vi "Create Sprite Points.vi"(4 "Scale":cluster{"X":sgl, "Y":sgl, "Z":sgl}, 5 "Sprite Type":T1=enum."Empty Square", 6 "Vertex Array":cluster{"X":sgl, "Y":sgl, "Z":sgl}[](array[cluster]), 7 "Point Size":sgl, 8 "error in (no error)":errorcluster, 9 "Index Array":i32[](array[numeric]), 10 "Color Array":cluster{"R":sgl, "G":sgl, "B":sgl, "A":sgl}[](array[cluster]), 11 "Dot Object In":refnum<vi>) -> (0 "error out":errorcluster, 3 "Dot Object Out":refnum<vi>)   [LabVIEW 2020, in "3D Plot.lvclass"]
uses:
  3D Plot.lvclass
  Sprite Type.ctl
  LV3DPointTypeDef.ctl
  NI_3D Picture Control.lvlib
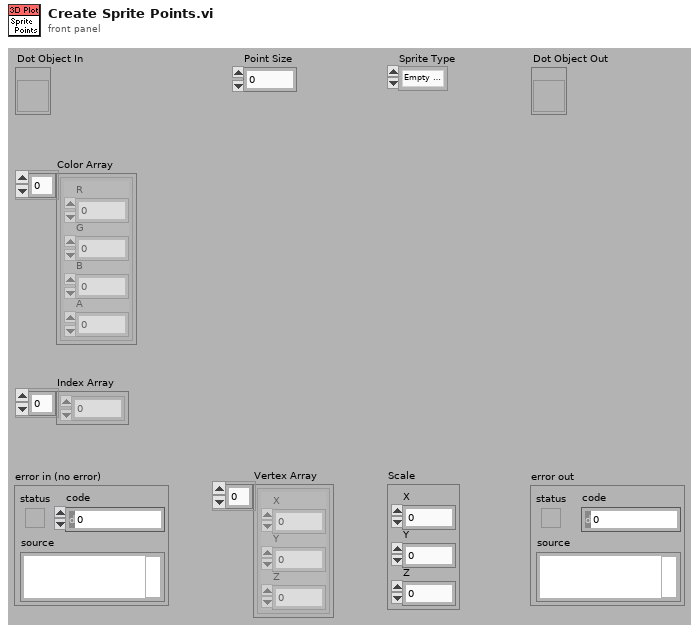
[diagram p1: front panel]
types:
  T1 = typedef "3D Plot.lvclass/Sprite Type.ctl" = enum16{"None", "Empty Square", "Solid Square", "Empty Diamond", "Solid Diamond", "Empty Circle", "Solid Circle", "Asterisk", "Bold X", "Wireframe Sphere", "Solid Sphere", "Wireframe Cube", "Solid Cube"}
  T2 = typedef "LV3DPointTypeDef.ctl" = cluster{"X":sgl, "Y":sgl, "Z":sgl}
  T3 = enum16{"Inherit Value", "Points", "Wireframe", "Polygons"}
  T4 = enum16{"Overall", "Per Primitive", "Per Vertex", "Binding Off"}
  T5 = enum16{"Points", "Lines", "Line Strip", "Line Loop", "Triangles", "Triangle Strip", "Triangle Fan", "Quads", "Quad Strip", "Polygon"}
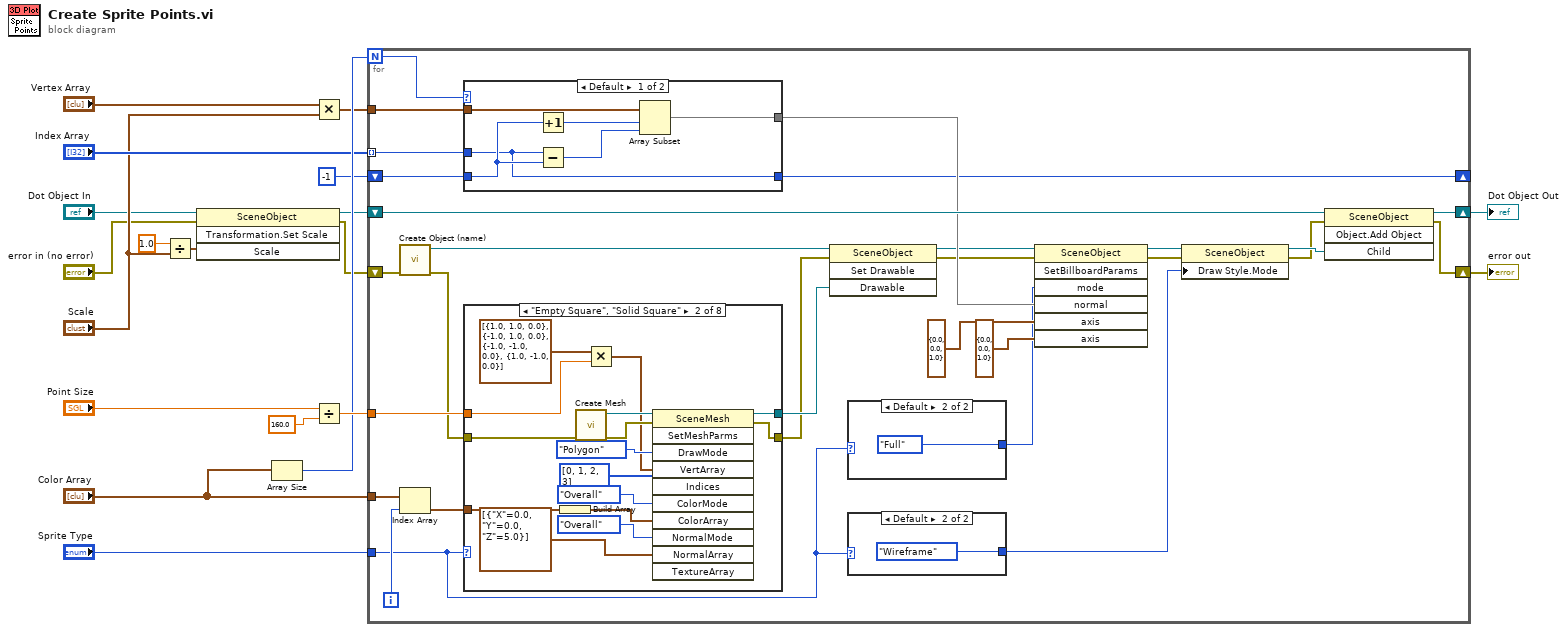
[diagram p0: block diagram]
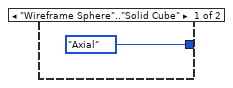
[diagram p2: hidden frame]
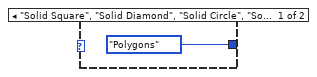
[diagram p4: hidden frame]
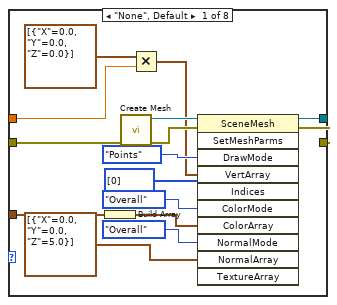
[diagram p5: hidden frame]
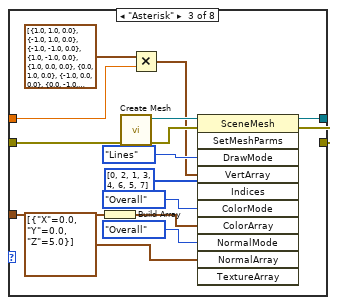
[diagram p6: hidden frame]
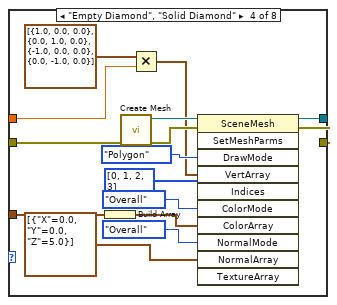
[diagram p7: hidden frame]
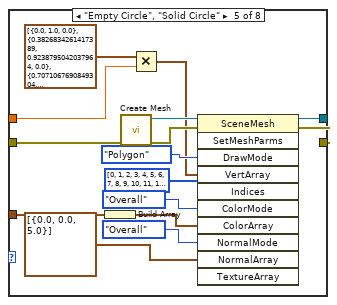
[diagram p8: hidden frame]
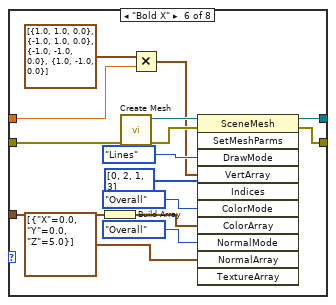
[diagram p9: hidden frame]
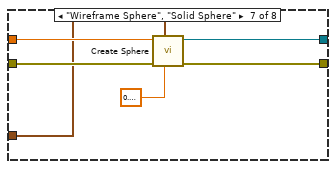
[diagram p10: hidden frame]
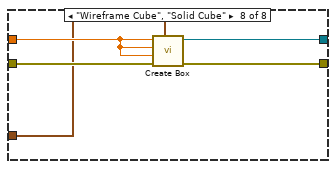
[diagram p11: hidden frame]
diagram:
  n1 = Divide(x=sgl 1.0, y="Scale") -> (x/y=w5:cluster{"X":sgl, "Y":sgl, "Z":sgl})
  n2 = invoke class="SceneObject" method="Transformation.Set Scale"(reference="Dot Object In", error in="error in (no error)", "Scale"=w5) -> (reference out=w3:refnum<vi>, error out=w1:errorcluster)  [unwired: 1 in, 2 out]
  n3 = Array Size(array="Color Array") -> (size(s)=w12:i32)
  n4 = Multiply(x="Vertex Array", y="Scale") -> (x*y=w7:cluster{"X":sgl, "Y":sgl, "Z":sgl}[])
  n5 = Divide(x="Point Size", y=sgl 160.0) -> (x/y=w16:sgl)
  n6 = for {
    N: w12 -> [w31]
    tunnel: "Color Array" -> [w48]
    tunnel: w16 -> [w47]
    tunnel: w7 -> [w30]
    tunnel: "Sprite Type" -> [w21]
    shift-right: [w33] -> w13
    shift-left: w3 -> [w34]
    shift-right: [w35] -> w15
    shift-left: w1 -> [w25]
    tunnel: "Index Array" -> [w28] mode=indexing
    shift-right: [w26] -> _
    shift-left: -1 -> [w27]
    i -> [w32]
    n7 = call "Create Object (name).vi"("error in (no error)"=w25) -> ("error out"=w38:errorcluster, "Scene:New Object"=w39:refnum<vi>)  [unwired: 9 in]
    n8 = Index Array(array=w48, index=w32) -> (element=w43:cluster{"R":sgl, "G":sgl, "B":sgl, "A":sgl})
    n9 = case shown="Default" w31 {
      tunnel: w30 -> [w56 w58]
      tunnel: [w55 w58] -> w29
      tunnel: w28 -> [w52 _]
      tunnel: w27 -> [w54 w57]
      tunnel: [w52 w57] -> w26
      frame Default {
        n10 = Increment(x=w54) -> (x+1=w51:i32)
        n11 = Subtract(x=w52, y=w54) -> (x-y=w53:i32)
        n12 = Array Subset(array=w56, index=w51, length=w53) -> (w55:cluster{"X":sgl, "Y":sgl, "Z":sgl}[])
      }
      frame 1 {
        # "All objects are in the same color, so create only one object and use Billborad \"pos list\" to form the remaining sprites in the plot."
      }
    }
    n13 = case shown="\"Empty Square\", \"Solid Square\"" w21 {
      tunnel: w38 -> [w66 w82 w98 w111 w127 w149 w156 w161]
      tunnel: [w64 w80 w97 w109 w126 w147 w155 w159] -> w41
      tunnel: w43 -> [w61 w76 w91 w106 w121 w136 w151 w157]
      tunnel: w47 -> [w67 w83 w99 w112 w128 w142 w154 w158]
      tunnel: [w65 w81 w96 w110 w125 w146 w153 w160] -> w42
      frame "None", Default {
        n14 = Build Array(w61) -> (w69:cluster{"R":sgl, "G":sgl, "B":sgl, "A":sgl}[])
        n15 = call "Create Mesh.vi"("error in (no error)"=w66) -> ("error out"=w74:errorcluster, "New Mesh Refnum"=w75:refnum<vi>)  [unwired: 9 out]
        n16 = Multiply(x=cluster{"X":sgl, "Y":sgl, "Z":sgl}[] [{"X"=0.0, "Y"=0.0, "Z"=0.0}] ("Vertex Array"), y=w67) -> (x*y=w71:cluster{"X":sgl, "Y":sgl, "Z":sgl}[])
        n17 = invoke class="SceneMesh" method="SetMeshParms"(reference=w75, error in=w74, "DrawMode"=T5."Points" ("Draw Mode"), "VertArray"=w71, "Indices"=u32[] [0], "ColorMode"=T4."Overall" ("Color Binding Mode"), "ColorArray"=w69, "NormalMode"=T4."Overall" ("Normal Binding Mode"), "NormalArray"=cluster{"X":sgl, "Y":sgl, "Z":sgl}[] [{"X"=0.0, "Y"=0.0, "Z"=5.0}] ("Vertex Array")) -> (reference out=w65:refnum<vi>, error out=w64:errorcluster)  [unwired: 2 in, 9 out]
      }
      frame "Empty Square", "Solid Square" {
        n18 = Build Array(w76) -> (w84:cluster{"R":sgl, "G":sgl, "B":sgl, "A":sgl}[])
        n19 = call "Create Mesh.vi"("error in (no error)"=w82) -> ("error out"=w89:errorcluster, "New Mesh Refnum"=w90:refnum<vi>)  [unwired: 9 out]
        n20 = Multiply(x=cluster{"X":sgl, "Y":sgl, "Z":sgl}[] [{"X"=1.0, "Y"=1.0, "Z"=0.0}, {"X"=-1.0, "Y"=1.0, "Z"=0.0}, {"X"=-1.0, "Y"=-1.0, "Z"=0.0}, {"X"=1.0, "Y"=-1.0, "Z"=0.0}] ("Vertex Array"), y=w83) -> (x*y=w86:cluster{"X":sgl, "Y":sgl, "Z":sgl}[])
        n21 = invoke class="SceneMesh" method="SetMeshParms"(reference=w90, error in=w89, "DrawMode"=T5."Polygon" ("Draw Mode"), "VertArray"=w86, "Indices"=u32[] [0, 1, 2, 3], "ColorMode"=T4."Overall" ("Color Binding Mode"), "ColorArray"=w84, "NormalMode"=T4."Overall" ("Normal Binding Mode"), "NormalArray"=cluster{"X":sgl, "Y":sgl, "Z":sgl}[] [{"X"=0.0, "Y"=0.0, "Z"=5.0}] ("Vertex Array")) -> (reference out=w81:refnum<vi>, error out=w80:errorcluster)  [unwired: 2 in, 9 out]
      }
      frame "Asterisk" {
        n22 = Build Array(w91) -> (w100:cluster{"R":sgl, "G":sgl, "B":sgl, "A":sgl}[])
        n23 = call "Create Mesh.vi"("error in (no error)"=w98) -> ("error out"=w104:errorcluster, "New Mesh Refnum"=w105:refnum<vi>)  [unwired: 9 out]
        n24 = Multiply(x=cluster{"X":sgl, "Y":sgl, "Z":sgl}[] [{"X"=1.0, "Y"=1.0, "Z"=0.0}, {"X"=-1.0, "Y"=1.0, "Z"=0.0}, {"X"=-1.0, "Y"=-1.0, "Z"=0.0}, {"X"=1.0, "Y"=-1.0, "Z"=0.0}, {"X"=1.0, "Y"=0.0, "Z"=0.0}, {"X"=0.0, "Y"=1.0, "Z"=0.0}, {"X"=-1.0, "Y"=0.0, "Z"=0.0}, {"X"=0.0, "Y"=-1.0, "Z"=0.0}] ("Vertex Array"), y=w99) -> (x*y=w101:cluster{"X":sgl, "Y":sgl, "Z":sgl}[])
        n25 = invoke class="SceneMesh" method="SetMeshParms"(reference=w105, error in=w104, "DrawMode"=T5."Lines" ("Draw Mode"), "VertArray"=w101, "Indices"=u32[] [0, 2, 1, 3, 4, 6, 5, 7], "ColorMode"=T4."Overall" ("Color Binding Mode"), "ColorArray"=w100, "NormalMode"=T4."Overall" ("Normal Binding Mode"), "NormalArray"=cluster{"X":sgl, "Y":sgl, "Z":sgl}[] [{"X"=0.0, "Y"=0.0, "Z"=5.0}] ("Vertex Array")) -> (reference out=w96:refnum<vi>, error out=w97:errorcluster)  [unwired: 2 in, 9 out]
      }
      frame "Empty Diamond", "Solid Diamond" {
        n26 = Build Array(w106) -> (w113:cluster{"R":sgl, "G":sgl, "B":sgl, "A":sgl}[])
        n27 = call "Create Mesh.vi"("error in (no error)"=w111) -> ("error out"=w119:errorcluster, "New Mesh Refnum"=w120:refnum<vi>)  [unwired: 9 out]
        n28 = Multiply(x=cluster{"X":sgl, "Y":sgl, "Z":sgl}[] [{"X"=1.0, "Y"=0.0, "Z"=0.0}, {"X"=0.0, "Y"=1.0, "Z"=0.0}, {"X"=-1.0, "Y"=0.0, "Z"=0.0}, {"X"=0.0, "Y"=-1.0, "Z"=0.0}] ("Vertex Array"), y=w112) -> (x*y=w115:cluster{"X":sgl, "Y":sgl, "Z":sgl}[])
        n29 = invoke class="SceneMesh" method="SetMeshParms"(reference=w120, error in=w119, "DrawMode"=T5."Polygon" ("Draw Mode"), "VertArray"=w115, "Indices"=u32[] [0, 1, 2, 3], "ColorMode"=T4."Overall" ("Color Binding Mode"), "ColorArray"=w113, "NormalMode"=T4."Overall" ("Normal Binding Mode"), "NormalArray"=cluster{"X":sgl, "Y":sgl, "Z":sgl}[] [{"X"=0.0, "Y"=0.0, "Z"=5.0}] ("Vertex Array")) -> (reference out=w110:refnum<vi>, error out=w109:errorcluster)  [unwired: 2 in, 9 out]
      }
      frame "Empty Circle", "Solid Circle" {
        n30 = Build Array(w121) -> (w129:cluster{"R":sgl, "G":sgl, "B":sgl, "A":sgl}[])
        n31 = call "Create Mesh.vi"("error in (no error)"=w127) -> ("error out"=w134:errorcluster, "New Mesh Refnum"=w135:refnum<vi>)  [unwired: 9 out]
        n32 = Multiply(x=cluster{sgl, sgl, sgl}[] [{0.0, 1.0, 0.0}, {0.38268343, 0.9238795, 0.0}, {0.70710677, 0.70710677, 0.0}, {0.9238795, 0.38268343, 0.0}, {1.0, 6.123032e-17, 0.0}, {0.9238795, -0.38268343, 0.0}, {0.70710677, -0.70710677, 0.0}, {0.38268343, -0.9238795, 0.0}, {1.2246064e-16, -1.0, 0.0}, {-0.38268343, -0.9238795, 0.0}, {-0.70710677, -0.70710677, 0.0}, {-0.9238795, -0.38268343, 0.0}, {-1.0, -1.8369095e-16, 0.0}, {-0.9238795, 0.38268343, 0.0}, {-0.70710677, 0.70710677, 0.0}, {-0.38268343, 0.9238795, 0.0}] ("Array"), y=w128) -> (x*y=w131:cluster{sgl, sgl, sgl}[])
        n33 = invoke class="SceneMesh" method="SetMeshParms"(reference=w135, error in=w134, "DrawMode"=T5."Polygon" ("Draw Mode"), "VertArray"=w131, "Indices"=u32[] [0, 1, 2, 3, 4, 5, 6, 7, 8, 9, 10, 11, 12, 13, 14, 15], "ColorMode"=T4."Overall" ("Color Binding Mode"), "ColorArray"=w129, "NormalMode"=T4."Overall" ("Normal Binding Mode"), "NormalArray"=cluster{sgl, sgl, sgl}[] [{0.0, 0.0, 5.0}] ("Array")) -> (reference out=w125:refnum<vi>, error out=w126:errorcluster)  [unwired: 2 in, 9 out]
      }
      frame "Bold X" {
        n34 = Build Array(w136) -> (w139:cluster{"R":sgl, "G":sgl, "B":sgl, "A":sgl}[])
        n35 = call "Create Mesh.vi"("error in (no error)"=w149) -> ("error out"=w148:errorcluster, "New Mesh Refnum"=w150:refnum<vi>)  [unwired: 9 out]
        n36 = Multiply(x=cluster{"X":sgl, "Y":sgl, "Z":sgl}[] [{"X"=1.0, "Y"=1.0, "Z"=0.0}, {"X"=-1.0, "Y"=1.0, "Z"=0.0}, {"X"=-1.0, "Y"=-1.0, "Z"=0.0}, {"X"=1.0, "Y"=-1.0, "Z"=0.0}] ("Vertex Array"), y=w142) -> (x*y=w141:cluster{"X":sgl, "Y":sgl, "Z":sgl}[])
        n37 = invoke class="SceneMesh" method="SetMeshParms"(reference=w150, error in=w148, "DrawMode"=T5."Lines" ("Draw Mode"), "VertArray"=w141, "Indices"=u32[] [0, 2, 1, 3], "ColorMode"=T4."Overall" ("Color Binding Mode"), "ColorArray"=w139, "NormalMode"=T4."Overall" ("Normal Binding Mode"), "NormalArray"=cluster{"X":sgl, "Y":sgl, "Z":sgl}[] [{"X"=0.0, "Y"=0.0, "Z"=5.0}] ("Vertex Array")) -> (reference out=w146:refnum<vi>, error out=w147:errorcluster)  [unwired: 2 in, 9 out]
      }
      frame "Wireframe Sphere", "Solid Sphere" {
        n38 = call "Create Sphere.vi"("Detail"=sgl 0.3, "Color"=w151, "error in (no error)"=w156, "Radius"=w154) -> ("error out"=w155:errorcluster, "New Sphere Refnum"=w153:refnum<vi>)  [unwired: 1 in, 5 out]
      }
      frame "Wireframe Cube", "Solid Cube" {
        n39 = call "Create Box.vi"("Color"=w157, "error in (no error)"=w161, "Length Z"=w158, "Length Y"=w158, "Length X"=w158) -> ("error out"=w159:errorcluster, "New Box Refnum"=w160:refnum<vi>)  [unwired: 5 out]
      }
    }
    n40 = invoke class="SceneObject" method="Set Drawable"(reference=w39, error in=w41, "Drawable"=w42) -> (reference out=w22:refnum<vi>, error out=w23:errorcluster)  [unwired: 1 in, 2 out]
    n41 = case shown="Default" w21 {
      tunnel: [enum16{"No Billboarding", "Axial", "Full"}."Axial" ("mode") enum16{"No Billboarding", "Axial", "Full"}."Full" ("mode")] -> w20
      frame "Wireframe Sphere".."Solid Cube" {
      }
      frame Default {
      }
    }
    n42 = case shown="Default" w21 {
      tunnel: [T3."Polygons" ("Draw Style:Mode") T3."Wireframe" ("Draw Style:Mode")] -> w40
      frame "Solid Square", "Solid Diamond", "Solid Circle", "Solid Sphere", "Solid Cube" {
      }
      frame Default {
      }
    }
    n43 = invoke class="SceneObject" method="SetBillboardParams"(reference=w22, error in=w23, "mode"=w20, "normal"=w29, "axis"=cluster{"X":sgl, "Y":sgl, "Z":sgl} {"X"=0.0, "Y"=0.0, "Z"=1.0} ("normal"), "axis"=T2 {"X"=0.0, "Y"=0.0, "Z"=1.0}) -> (reference out=w45:refnum<vi>, error out=w44:errorcluster)  [unwired: 1 in, 5 out]
    n44 = property class="SceneObject"(reference=w45, error in=w44, "Draw Style.Mode"=w40) -> (reference out=w37:refnum<vi>, error out=w36:errorcluster)
    n45 = invoke class="SceneObject" method="Object.Add Object"(reference=w34, error in=w36, "Child"=w37) -> (reference out=w33:refnum<vi>, error out=w35:errorcluster)  [unwired: 1 in, 2 out]
  }
  "Dot Object Out" <- w13
  "error out" <- w15
